vi "Tx Timestamp Channel Page.vi"(8 "error in (no error)":errorcluster, 11 "Node Ptr":T1 format="%.0x") -> (0 "error out":errorcluster)   [LabVIEW 2019]
uses:
  <vilib>/NI VeriStand/Custom Device API/Custom Device Item Ref.ctl
  <vilib>/NI VeriStand/Custom Device API/Custom Device API.lvlib
  UDP-Custom-Device System Explorer.lvlib
panel:
  in  "SHDocVw.IWebBrowser":refnum<k7>(container)
  in  "General Header":cluster{"Section Name":string}={"Section Name"="Tx Timestamp Channel"}
  in  "Description":string
  out "Name":string
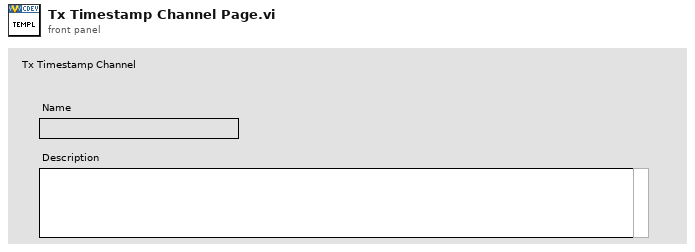
[diagram p1: front panel]
types:
  T1 = typedef "Custom Device API.lvlib/Custom Device Item Ref.ctl" = u64
  T2 = typedef "Custom Device API.lvlib/Custom Device Item Info.ctl" = cluster{"Name":string, "Is Channel":bool, "GUID":string, "Is Waveform":bool}
  T3 = typedef "Custom Device API.lvlib/Custom Device Commands.ctl" = enum16{"Default", "Item renamed", "Shutdown", "Dynamic button pressed"}
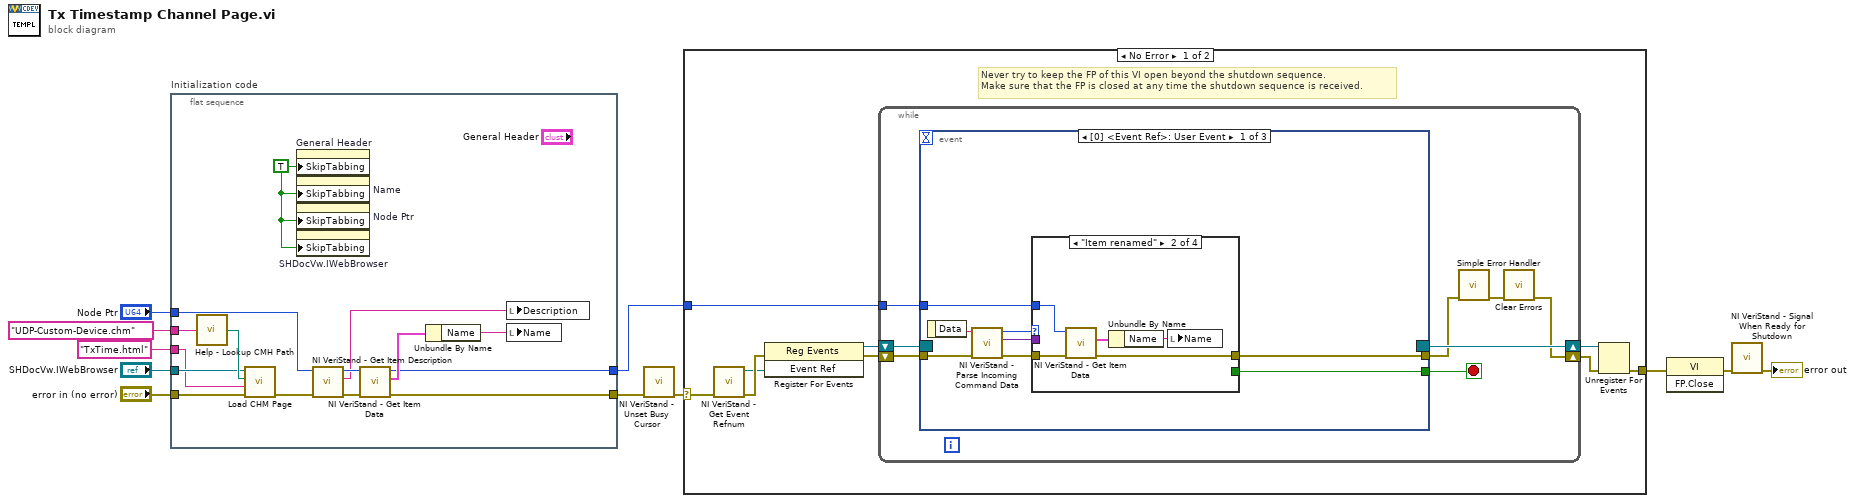
[diagram p0: block diagram]
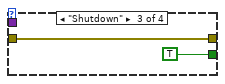
[diagram p3: hidden frame]
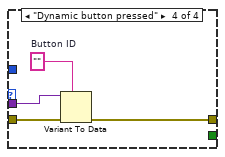
[diagram p4: hidden frame]
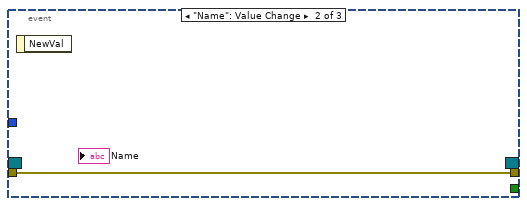
[diagram p5: hidden frame]
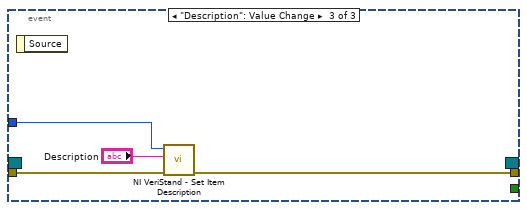
[diagram p6: hidden frame]
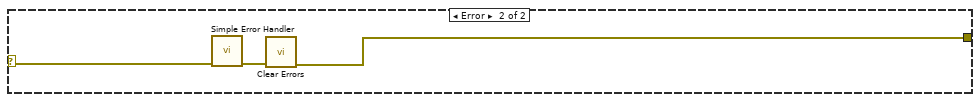
[diagram p7: hidden frame]
diagram:
  n1 = flat-sequence "Initialization code" {
    tunnel: "error in (no error)" -> [w19]
    tunnel: "Node Ptr" -> [w23]
    tunnel: [w14] -> w7
    tunnel: [w13] -> w4
    tunnel: "SHDocVw.IWebBrowser" -> [w17]
    tunnel: "TxTime.html" ("CD_CHM_Section") -> [w16]
    tunnel: "UDP-Custom-Device.chm" ("CD_CHM_FileName") -> [w18]
    frame #0 {
      w12 = TRUE ("Skip When Tabbing")
      n2 = call "Help - Lookup CMH Path.vi"("Main CMH File"=w18) -> ("Compiled CMH Path"=w20:path)
      n3 = call <vilib>:"Load CHM Page.vi"("error in (no error)"=w19, "HTML File"=w16, "Compiled CHM Path"=w20, "Web Browser Reference"=w17) -> ("error out"=w15:errorcluster)  [unwired: 7 in]
      n4 = property on="General Header" class="Clust (strict)"("SkipTabbing"=w12) -> ()  [unwired: 2 in, 2 out]
      n5 = property on="Name" class="Str"("SkipTabbing"=w12) -> ()  [unwired: 2 in, 2 out]
      n6 = property on="Node Ptr" class="DigNum (strict)"("SkipTabbing"=w12) -> ()  [unwired: 2 in, 2 out]
      n7 = property on="SHDocVw.IWebBrowser" class="AXCont"("SkipTabbing"=w12) -> ()  [unwired: 2 in, 2 out]
      n8 = call <vilib>:"NI VeriStand - Get Item Description.vi"("error in (no error)"=w15, "Item Ref in"=w23) -> ("error out"=w25:errorcluster, "Description"=w21:string, "Item Ref out"=w26:T1)  [unwired: 7 out]
      n9 = call <vilib>:"NI VeriStand - Get Item Data.vi"("error in (no error)"=w25, "Item Ref in"=w26) -> ("error out"=w14:errorcluster, "Item Info"=w24:T2, "Item Ref out"=w13:T1)  [unwired: 7 out]
      n10 = Unbundle By Name(w24) -> ("Name"=w22:string)
      n11 = local write "Description"(w21) -> ()
      n12 = local write "Name"(w22) -> ()
    }
  }
  n13 = call <vilib>:"NI VeriStand - Unset Busy Cursor.vi"("error in (no error)"=w7) -> ("error out"=w6:errorcluster)  [unwired: 10 out]
  n14 = case shown="No Error" w6 {
    selector: w6 -> [w27 w71]
    tunnel: [w32 w69] -> w11
    tunnel: w4 -> [w28 _]
    frame No Error {
      # "Never try to keep the FP of this VI open beyond the shutdown sequence.\nMake sure that the FP is closed at any time the shutdown sequence is received."
      n15 = call <vilib>:"NI VeriStand - Get Event Refnum.vi"("error in (no error)"=w27) -> ("error out"=w35:errorcluster, "Event Ref"=w31:refnum<user-event>)  [unwired: 9 out]
      n16 = register-events(error in=w35, w31) -> (reference out=w29:refnum<event-registration>, error out=w30:errorcluster)  [unwired: 1 in]
      n17 = while {
        tunnel: w28 -> [w39]
        shift-right: [w36] -> w33
        shift-left: w30 -> [w42]
        shift-right: [w43] -> w34
        shift-left: w29 -> [w41]
        stop <- w40 stop-if-true
        n18 = event shown="[0] <Event Ref>: User Event" {
          selector: w41 -> [_ _ _]
          dyn-events: [_ _ _] -> w43
          timeout: _ -> [_ _ _]
          tunnel: w42 -> [w51 w64 w67]
          tunnel: [w47 _ _] -> w40
          tunnel: [w46 w64 w66] -> w38
          tunnel: w39 -> [w45 _ w68]
          event User Event {
            n19 = event-data() -> ("Data"=w50:string)  [unwired: 1 out]
            n20 = call <vilib>:"NI VeriStand - Parse Incoming Command Data.vi"("error in (no error)"=w51, "Incoming data"=w50) -> ("error out"=w49:errorcluster, "Outgoing data"=w44:variant, "Action"=w48:T3)  [unwired: 7 out]
            n21 = case shown="\"Item renamed\"" w48 {
              tunnel: w49 -> [w52 w57 w58 w63]
              tunnel: [_ _ TRUE _] -> w47
              tunnel: [w52 w54 w58 w60] -> w46
              tunnel: w45 -> [_ w56 _ _]
              tunnel: w44 -> [_ _ _ w62]
              frame "Default", Default {
              }
              frame "Item renamed" {
                n22 = call <vilib>:"NI VeriStand - Get Item Data.vi"("error in (no error)"=w57, "Item Ref in"=w56) -> ("error out"=w54:errorcluster, "Item Info"=w55:T2)  [unwired: 8 out]
                n23 = Unbundle By Name(w55) -> ("Name"=w53:string)
                n24 = local write "Name"(w53) -> ()
              }
              frame "Shutdown" {
              }
              frame "Dynamic button pressed" {
                w61 = ""  # Button ID
                n25 = Variant To Data(error in=w63, type=w61, Variant=w62) -> (error out=w60:errorcluster)  [unwired: 1 out]
              }
            }
          }
          event "Name": Value Change {
            n26 = event-data() -> ()  [unwired: 2 out]
          }
          event "Description": Value Change {
            n27 = event-data() -> ()  [unwired: 2 out]
            n28 = call <vilib>:"NI VeriStand - Set Item Description.vi"("error in (no error)"=w67, "Description"="Description", "Item Ref in"=w68) -> ("error out"=w66:errorcluster)  [unwired: 8 out]
          }
        }
        n29 = call <vilib>:"Simple Error Handler.vi"("error in (no error)"=w38) -> ("error out"=w37:errorcluster)  [unwired: 1 in, 7 out]
        n30 = call <vilib>:"Clear Errors.vi"("error in (no error)"=w37) -> ("error out"=w36:errorcluster)  [unwired: 1 in, 5 out]
      }
      n31 = Unregister For Events(event registration refnum=w34, error in=w33) -> (error out=w32:errorcluster)
    }
    frame Error {
      n32 = call <vilib>:"Simple Error Handler.vi"("error in (no error)"=w71) -> ("error out"=w70:errorcluster)  [unwired: 1 in, 7 out]
      n33 = call <vilib>:"Clear Errors.vi"("error in (no error)"=w70) -> ("error out"=w69:errorcluster)  [unwired: 1 in, 5 out]
    }
  }
  n34 = invoke class="VI" method="FP.Close"(error in=w11) -> (error out=w10:errorcluster)  [unwired: 2 in, 2 out]
  n35 = call <vilib>:"NI VeriStand - Signal When Ready for Shutdown.vi"("error in (no error)"=w10) -> ("error out"=→"error out":errorcluster)  [unwired: 10 out]
